vi "Shared Set Object Pointer.vi"(10 "Object Pointer":i64, 11 "TreeNodeArray in":refnum<class "TreeNodeArray.lvclass">) -> (3 "TreeNodeArray out":refnum<class "TreeNodeArray.lvclass">)   [LabVIEW 2013, in "MDSplus.lvlib" / "TreeNodeArray.lvclass"]
uses:
  <vilib>/MDSplus/Classes/TreeNodeArray_Class/TreeNodeArray.lvclass
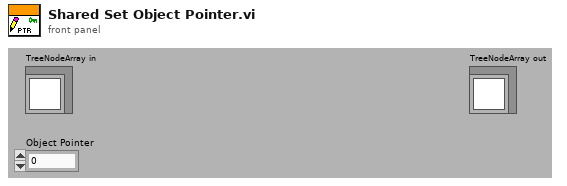
[diagram p1: front panel]
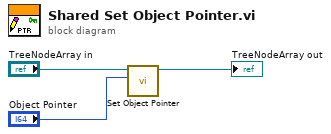
[diagram p0: block diagram]
diagram:
  n1 = call-dynamic "Set Object Pointer.vi"("Object Pointer"="Object Pointer", "TreeNodeArray in"="TreeNodeArray in") -> ("TreeNodeArray out"=→"TreeNodeArray out":refnum<class "TreeNodeArray.lvclass">)  [unwired: 9 in]
